vi "Check xls cloumn element.vi"(8 "code":string, 10 "name":string, 11 "file path (dialog if empty)":path caption="文件路径 （空时为对话框）") -> (3 "repeat？":bool)   [LabVIEW 2018]
uses:
  <vilib>/Utility/file.llb/Read Delimited Spreadsheet (string).vi
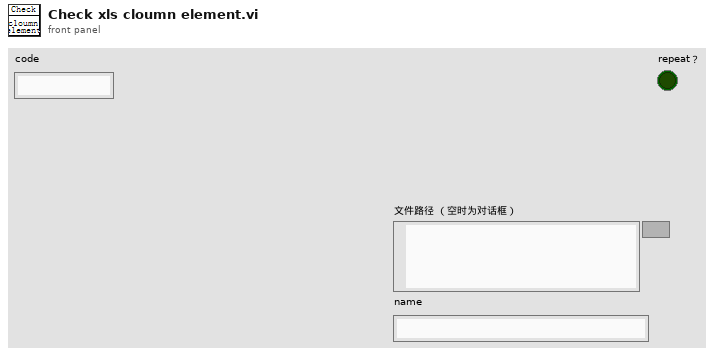
[diagram p1: front panel]
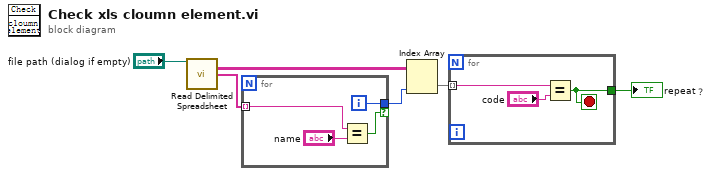
[diagram p0: block diagram]
diagram:
  n1 = call-poly <vilib>:"Read Delimited Spreadsheet.vi"("file path (dialog if empty)"="file path (dialog if empty)") -> ("all rows"=w4:string[][], "first row"=w5:string[])  [unwired: 9 in, 4 out]
  n2 = for {
    tunnel: w5 -> [w10] mode=indexing
    tunnel: [w8] -> w3 if=w7
    i -> [w8]
    n3 = Equal?(x=w10, y="name") -> (x = y?=w7:bool)
  }
  n4 = Index Array(array=w4, index (col)=w3) -> (element=w2:string[])  [unwired: 1 in]
  n5 = for {
    tunnel: w2 -> [w13] mode=indexing
    tunnel: [w11] -> w1
    stop <- w11 stop-if-true
    n6 = Equal?(x=w13, y="code") -> (x = y?=w11:bool)
  }
  "repeat？" <- w1
